vi "Scan_ver2_2.vi"(0 "DMM ref":refnum<visa-resource-name>, 1 "output cluster":cluster{"y":i32, i32, "Sample number":i32}={"y"=0, 0, "Sample number"=1}, 2 "P_current_count":i32, 3 "N_current_count":i32, 5 "DMM error":errorcluster, 7 "Current Sense \nResitance Array":dbl[](array[numeric])=[1.0032214, 1.00250644, 1.00234822, 1.0040944, 1.0017711, 1.00229431, 1.00344206, 1.00482066, 1.00381056, 1.00290978, 1.00333016, 1.00367587], 9 "ESP32 ref":refnum<visa-resource-name>, 11 "ESP32 error":errorcluster, 12 "current_mode":u8[](array[numeric])=[0, 0, 0, 0, 0, 0, 0, 0, 0, 0, 0]) -> (4 "DMM ref":refnum<visa-resource-name>, 6 "DMM error":errorcluster, 8 "Measurements":dbl[](array[numeric]), 10 "ESP32 ref":refnum<visa-resource-name>, 13 "Timout?":bool, 14 "Time out count":i32, 15 "ESP32 error":errorcluster)   [LabVIEW 2023]
uses:
  <instrlib>/Agilent 3446X Series/Agilent 3446X Series.lvlib
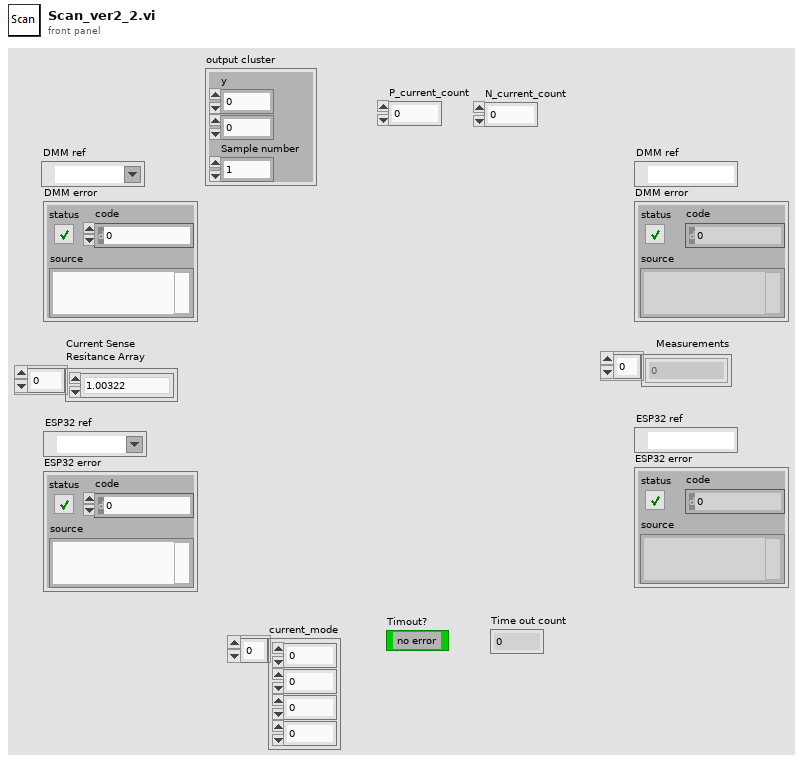
[diagram p1: front panel]
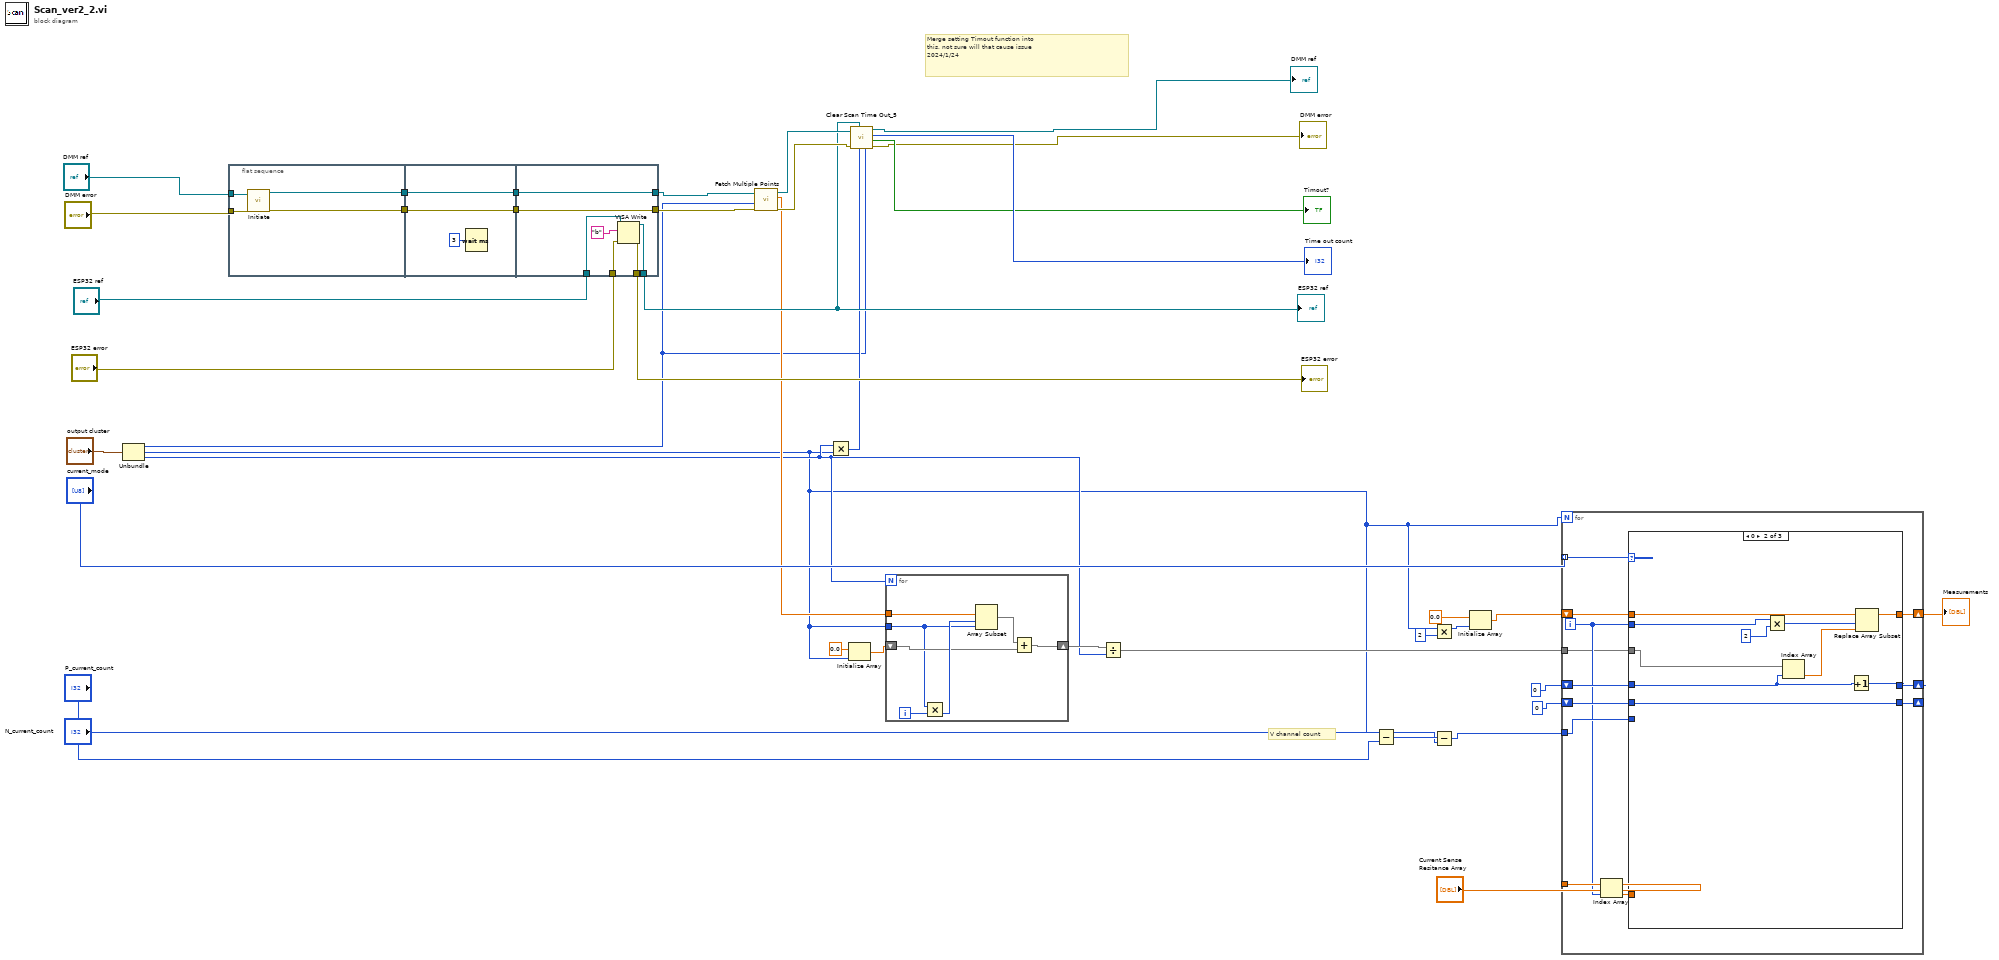
[diagram p0: block diagram]
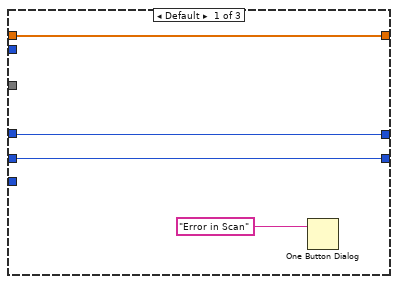
[diagram p2: hidden frame]
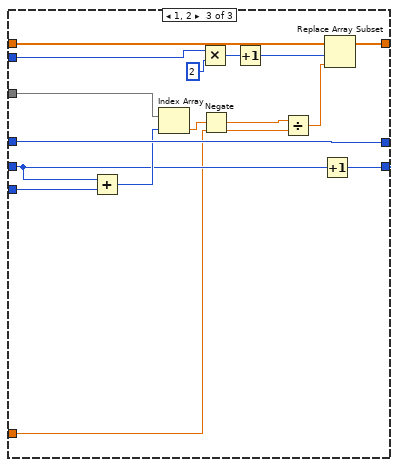
[diagram p3: hidden frame]
diagram:
  # "Merge setting Timout function into\nthis, not sure will that cause issue\n2024/1/24"
  # "V channel count"
  n1 = Unbundle("output cluster") -> ("y"=w3:i32, w4:i32, "Sample number"=w5:i32)
  n2 = flat-sequence {
    tunnel: [w45] -> w41
    tunnel: [w44] -> w40
    tunnel: "DMM ref" -> [w43]
    tunnel: "DMM error" -> [w42]
    tunnel: w41 -> [w48]
    tunnel: [w48] -> w39
    tunnel: w40 -> [w47]
    tunnel: [w47] -> w38
    tunnel: w39 -> [w55]
    tunnel: w38 -> [w54]
    tunnel: "ESP32 ref" -> [w53]
    tunnel: "ESP32 error" -> [w52]
    tunnel: [w51] -> w30
    tunnel: [w50] -> w31
    tunnel: [w55] -> w15
    tunnel: [w54] -> w14
    frame #0 {
      n3 = call <instrlib>:"Initiate.vi"("error in (no error)"=w42, "VISA resource name"=w43) -> ("error out"=w45:errorcluster, "VISA resource name out"=w44:refnum<visa-resource-name>)  [unwired: 8 in]
    }
    frame #1 {
      n4 = Wait (ms)(milliseconds to wait=u32 3) -> ()  [unwired: 1 out]
    }
    frame #2 {
      n5 = VISA Write(VISA resource name=w53, write buffer="b" ("data in"), error in (no error)=w52) -> (VISA resource name out=w51:refnum<visa-resource-name>, error out=w50:errorcluster)  [unwired: 1 out]
    }
  }
  n6 = call <instrlib>:"Fetch Multiple Points.vi"("error in (no error)"=w15, "Timeout (10000 ms)"=w3, "VISA resource name"=w14) -> ("error out"=w36:errorcluster, "Measurements"=w10:dbl[], "VISA resource name out"=w37:refnum<visa-resource-name>)  [unwired: 1 in, 5 out]
  n7 = Multiply(x=w5, y=w4) -> (x*y=w6:i32)
  n8 = Initialize Array(0.0 ("element"), w4) -> (w9:dbl[])
  n9 = call "Clear Scan Time Out_5.vi"("Timeout"=w3, "Channel number\nx Sample number"=w6, "ESP32 ref"=w30, "error in (no error)"=w36, "VISA Refnum in"=w37) -> ("error out"=→"DMM error":errorcluster, "error?"=→"Timout?":bool, "Time out count"=→"Time out count":i32, "VISA Refnum out"=→"DMM ref":refnum<visa-resource-name>)  [unwired: 2 in, 1 out]
  n10 = for {
    N: w5 -> [_]
    tunnel: w10 -> [w60]
    shift-right: [w57] -> w8
    shift-left: w9 -> [w58]
    tunnel: w4 -> [w56]
    i -> [w62]
    n11 = Multiply(x=w56, y=w62) -> (x*y=w61:i32)
    n12 = Array Subset(array=w60, index=w61, length=w56) -> (w59:dbl[])
    n13 = Add(x=w59, y=w58) -> (x+y=w57:dbl[])
  }
  n14 = Divide(x=w8, y=w5) -> (x/y=w7:dbl[])
  n15 = Subtract(x=w4, y="P_current_count") -> (x-y=w22:i32)
  n16 = Multiply(x=w4, y=2) -> (x*y=w26:i32)
  n17 = Subtract(x=w22, y="N_current_count") -> (x-y=w12:i32)
  n18 = Initialize Array(0.0 ("Measurement"), w26) -> (w24:dbl[])
  n19 = for {
    N: w4 -> [_]
    shift-right: [w70] -> w17
    shift-left: w24 -> [w71]
    tunnel: "current_mode" -> [w74] mode=indexing
    tunnel: w12 -> [w67]
    shift-right: [w72] -> _
    shift-left: 0 ("index") -> [w73]
    shift-right: [w68] -> _
    shift-left: 0 ("index") -> [w69]
    tunnel: "Current Sense \nResitance Array" -> [w66]
    tunnel: w7 -> [w63]
    i -> [w65]
    n20 = Index Array(array=w66, index=w65) -> (element=w64:dbl)
    n21 = case shown="0" w74 {
      tunnel: w73 -> [w78 w88 w98]
      tunnel: [w78 w87 w98] -> w72
      tunnel: w65 -> [_ w85 w103]
      tunnel: w71 -> [w77 w86 w104]
      tunnel: [w77 w83 w100] -> w70
      tunnel: w69 -> [w76 w82 w95]
      tunnel: [w76 w82 w94] -> w68
      tunnel: w67 -> [_ _ w97]
      tunnel: w64 -> [_ _ w92]
      tunnel: w63 -> [_ w80 w90]
      frame Default {
        n22 = One Button Dialog(message="Error in Scan") -> ()  [unwired: 1 in, 1 out]
      }
      frame 0 {
        n23 = Multiply(x=w85, y=2 ("x")) -> (x*y=w81:i32)
        n24 = Index Array(array=w80, index=w88) -> (element=w79:dbl)
        n25 = Increment(x=w88) -> (x+1=w87:i32)
        n26 = Replace Array Subset(array=w86, new element=w79, index=w81) -> (w83:dbl[])
      }
      frame 1, 2 {
        n27 = Add(x=w95, y=w97) -> (x+y=w96:i32)
        n28 = Index Array(array=w90, index=w96) -> (element=w89:dbl)
        n29 = Multiply(x=w103, y=2 ("x")) -> (x*y=w101:i32)
        n30 = Negate(x=w89) -> (-x=w91:dbl)
        n31 = Increment(x=w101) -> (x+1=w99:i32)
        n32 = Divide(x=w91, y=w92) -> (x/y=w93:dbl)
        n33 = Increment(x=w95) -> (x+1=w94:i32)
        n34 = Replace Array Subset(array=w104, new element=w93, index=w99) -> (w100:dbl[])
      }
    }
  }
  "Measurements" <- w17
  "ESP32 ref" <- w30
  "ESP32 error" <- w31
